vi "Test Test Pass if Expected API Call Made Using Tolerant Comparator.vi"(8 "error in (no error)":errorcluster, 11 "Test Case In":refnum<class "One Expectation Test.lvclass">) -> (0 "error out":errorcluster, 3 "Test Case Out":refnum<class "One Expectation Test.lvclass">)   [LabVIEW 2020, in "One Expectation Test.lvclass"]
uses:
  One Expectation Test.lvclass
  C:/Program Files (x86)/National Instruments/LabVIEW 2020/vi.lib/Astemes/LUnit/Test Case.lvclass
  Test Doubles/Test Interface Responsive Mock/Test Interface Mock.lvclass
  C:/git/astemes-lmock/source/Framework/Mock/Mock.lvclass
  source/Expectations/One/One Tolerant Inputs.vi
  Expectation Test/Expectation Test.lvclass
  source/Framework/LMock API.lvlib
  source/Expectations/One/One.lvlib
  C:/git/astemes-lmock/tests/Test Doubles/Test Interface Responsive Mock/Test Interface Mock.lvclass
  C:/git/astemes-lmock/tests/Test Doubles/Test Interface/Test Interface.lvclass
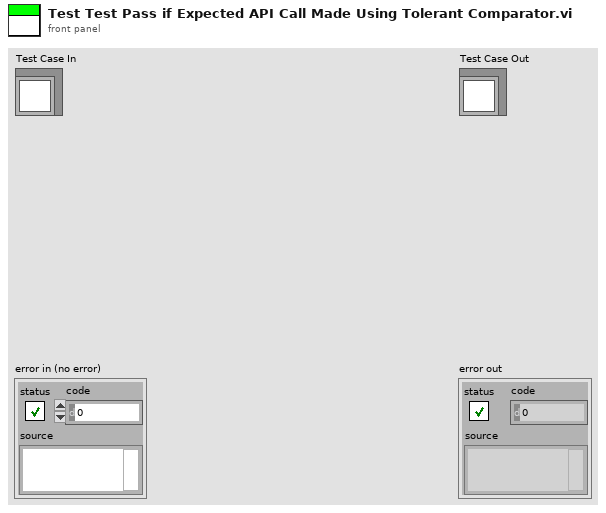
[diagram p1: front panel]
types:
  T1 = enum16{"", "Passed", "Failed", "Error", "Skipped", "Setup Error", "Broken", "Teardown Error"}
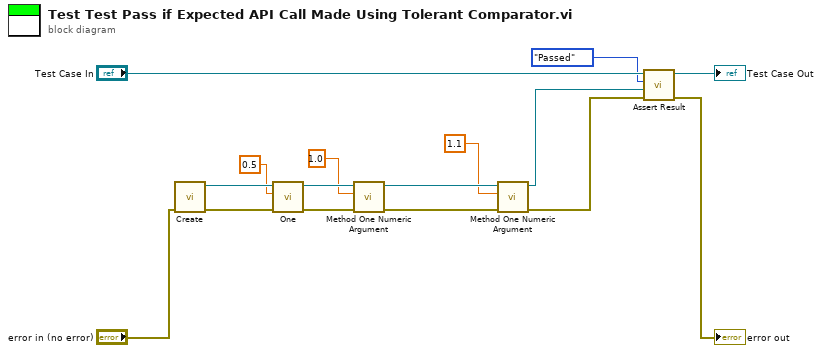
[diagram p0: block diagram]
diagram:
  n1 = call "Create.vi"("error in (no error)"="error in (no error)") -> ("error out"=w15:errorcluster, "Test Interface Mock Out"=w16:refnum<class "Test Interface Mock.lvclass">)  [unwired: 9 in]
  n2 = call-poly "One.vi"("error in (no error)"=w15, "Tolerance"=0.5, "Mock in"=w16) -> ("error out"=w13:errorcluster, "Mock out"=w14:refnum<class "Test Interface Mock.lvclass">)  [unwired: 7 in]
  n3 = call-dynamic "Method One Numeric Argument.vi"("error in (no error)"=w13, "Numeric"=1.0, "Test Interface Mock In"=w14) -> ("error out"=w12:errorcluster, "Test Interface Mock Out"=w5:refnum<class "Test Interface Mock.lvclass">)  [unwired: 7 in]
  n4 = call-dynamic "Method One Numeric Argument.vi"("error in (no error)"=w12, "Numeric"=1.1, "Test Interface Mock In"=w5) -> ("error out"=w6:errorcluster, "Test Interface Mock Out"=w4:refnum<class "Test Interface Mock.lvclass">)  [unwired: 7 in]
  n5 = call "Assert Result.vi"("error in (no error)"=w6, "Mock"=w4, "Status"=T1."Passed", "LUnit Test Case In"="Test Case In") -> ("error out"=→"error out":errorcluster, "LUnit Test Case Out"=→"Test Case Out":refnum<class "One Expectation Test.lvclass">)  [unwired: 6 in]
